vi "Comparación con matriz.vi"() -> ()   [LabVIEW 2016]
panel:
  out "Array 4":bool[][](array[boolean])
  out "Array 3":bool[](array[boolean])
  out "x > y?":bool
  out "Numeric Control":dbl
  out "Array 2":dbl[](array[numeric])
  in  "Array":dbl[][](array[numeric])
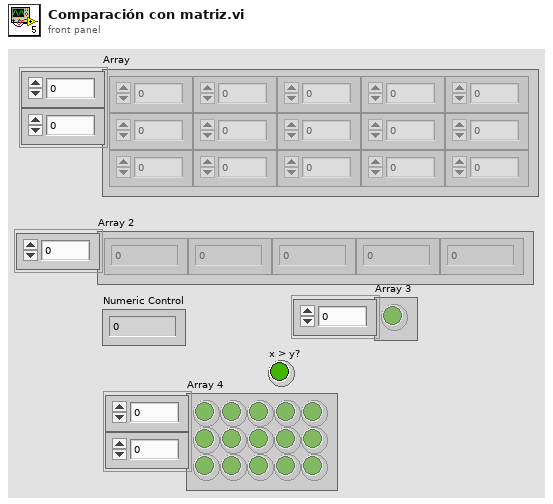
[diagram p1: front panel]
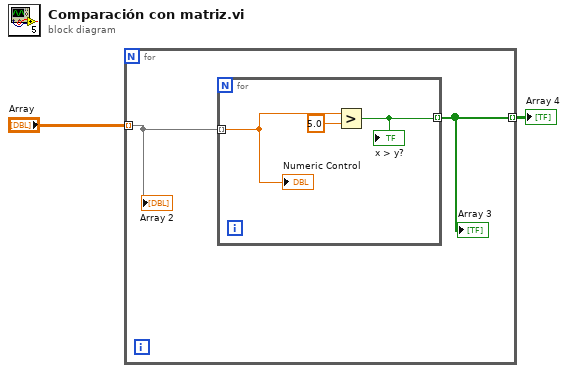
[diagram p0: block diagram]
diagram:
  n1 = for {
    tunnel: "Array" -> [w4] mode=indexing
    tunnel: [w3] -> w1 mode=indexing
    n2 = for {
      tunnel: w4 -> [w7] mode=indexing
      tunnel: [w5] -> w3 mode=indexing
      n3 = Greater?(x=w7, y=5.0) -> (0:w5:bool)
      "x > y?" <- w5
      "Numeric Control" <- w7
    }
    "Array 3" <- w3
    "Array 2" <- w4
  }
  "Array 4" <- w1
